vi "large-object-count-test.vi"(8 "error in (no error)":errorcluster) -> (0 "error out":errorcluster)   [LabVIEW 2013]
uses:
  src/SMO/SMO.lvclass
  <vilib>/addons/_JKI Toolkits/Caraya/classes/Test/Test.lvclass
  <vilib>/addons/_JKI Toolkits/Caraya/classes/Assert/Assert.lvclass
panel:
  out "Total Time":dbl
  out "destroy":i32
  out "stop":i32
  out "start":i32
  out "create":i32
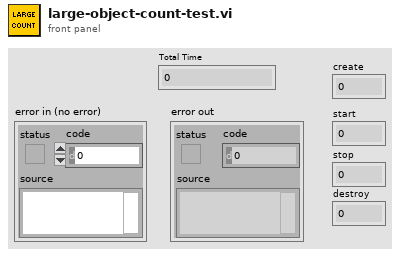
[diagram p1: front panel]
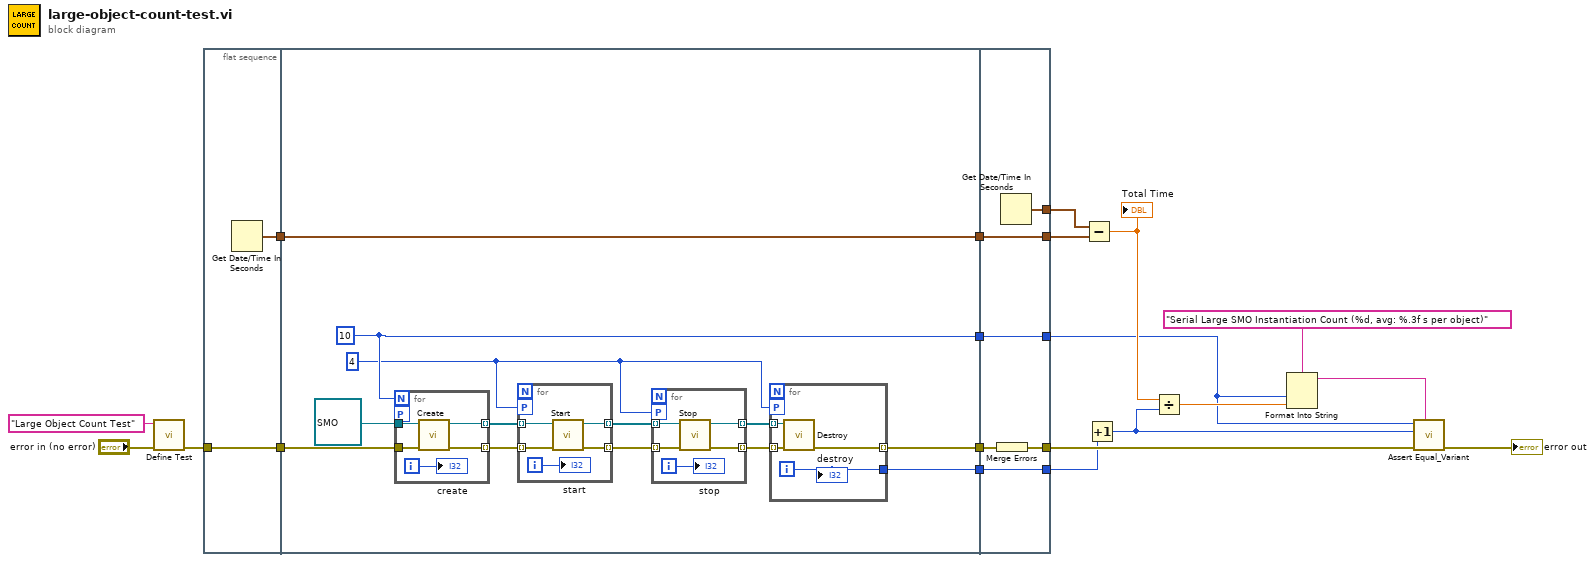
[diagram p0: block diagram]
diagram:
  n1 = call <vilib>:"Define Test.vi"("error in (no error)"="error in (no error)", "Label (VI Title)"="Large Object Count Test") -> ("error out"=w18:errorcluster)  [unwired: 9 in]
  n2 = flat-sequence {
    tunnel: w18 -> [w22]
    tunnel: [w22] -> w9
    tunnel: [w21] -> w4
    tunnel: w9 -> [w34]
    tunnel: [w33] -> w8
    tunnel: [w25] -> w7
    tunnel: [w26] -> w5
    tunnel: w4 -> [w26]
    tunnel: [w24] -> w1
    tunnel: [w59] -> w10
    tunnel: [w56] -> w17
    tunnel: w8 -> [w60]
    tunnel: w7 -> [w59]
    tunnel: [w58] -> w6
    tunnel: w5 -> [w58]
    tunnel: [w57] -> w3
    tunnel: [w55] -> w2
    tunnel: w1 -> [w55]
    frame #0 {
      n3 = Get Date/Time In Seconds() -> (seconds since 1Jan1904=w21:timestamp)
    }
    frame #1 {
      w23 = 4
      w25 = 10
      n4 = for {
        N: w25 -> [_]
        tunnel: refnum<class "SMO.lvclass"> refnum ("SMO.lvclass") -> [w54]
        tunnel: w34 -> [w53]
        tunnel: [w52] -> w30 mode=indexing
        tunnel: [w51] -> w29 mode=indexing
        workers-P: _ -> [_]
        i -> [w50]
        n5 = call "Create.vi"("error in (no error)"=w53, "SMO"=w54) -> ("error out"=w51:errorcluster, "SMO out"=w52:refnum<class "SMO.lvclass">)  [unwired: 7 in, 1 out]
        "create" <- w50
      }
      n6 = for {
        tunnel: w30 -> [w49] mode=indexing
        tunnel: w29 -> [w48] mode=indexing
        tunnel: [w47] -> w28 mode=indexing
        tunnel: [w46] -> w27 mode=indexing
        workers-P: w23 -> [_]
        i -> [w45]
        n7 = call "Start.vi"("error in (no error)"=w48, "SMO"=w49) -> ("error out"=w46:errorcluster, "SMO out"=w47:refnum<class "SMO.lvclass">)  [unwired: 8 in]
        "start" <- w45
      }
      n8 = for {
        tunnel: [w44] -> w32 mode=indexing
        tunnel: [w43] -> w31 mode=indexing
        tunnel: w28 -> [w42] mode=indexing
        tunnel: w27 -> [w41] mode=indexing
        workers-P: w23 -> [_]
        i -> [w40]
        n9 = call "Stop.vi"("error in (no error)"=w41, "SMO"=w42) -> ("error out"=w44:errorcluster, "SMO out"=w43:refnum<class "SMO.lvclass">)  [unwired: 8 in]
        "stop" <- w40
      }
      n10 = for {
        tunnel: [w39] -> w33 mode=indexing
        tunnel: w32 -> [w38] mode=indexing
        tunnel: w31 -> [w37] mode=indexing
        tunnel: [w36] -> w24
        workers-P: w23 -> [_]
        i -> [w36]
        n11 = call "Destroy.vi"("error in (no error)"=w38, "SMO"=w37) -> ("error out"=w39:errorcluster)  [unwired: 9 in]
        "destroy" <- w36
      }
    }
    frame #2 {
      n12 = Merge Errors(w60) -> (w56:errorcluster)
      n13 = Get Date/Time In Seconds() -> (seconds since 1Jan1904=w57:timestamp)
    }
  }
  n14 = Subtract(x=w3, y=w6) -> (x-y=w15:dbl)
  "Total Time" <- w15
  n15 = Increment(x=w2) -> (x+1=w14:i32)
  n16 = Divide(x=w15, y=w14) -> (x/y=w13:dbl)
  n17 = Format Into String(format string="Serial Large SMO Instantiation Count (%d, avg: %.3f s per object)" ("Label"), w10, w13) -> (resulting string=w12:string)  [unwired: 2 in, 1 out]
  n18 = call <vilib>:"Assert Equal_Variant.vi"("Label"=w12, "error in (no error)"=w17, "Y"=w14, "X"=w10) -> ("error out"=→"error out":errorcluster)  [unwired: 7 in]
